vi "To Serial Form.vi"(6 "Serial Version":T1, 10 "Serializer in":refnum<class "Serializer.lvclass">, 11 "BrowerComponent in":refnum<class "BrowerComponent.lvclass">) -> (0 "error out":errorcluster, 2 "Serializer out":refnum<class "Serializer.lvclass">, 3 "BrowerComponent out":refnum<class "BrowerComponent.lvclass">)   [LabVIEW 2015, in "BrowerComponent.lvclass"]
uses:
  BrowerComponent.lvclass
  <vilib>/NI/AQ Character Lineator/Serializer/Serializer.lvclass
  <vilib>/NI/AQ Character Lineator/Serialization Common/Serial Version.ctl
  protected/ObjectAttributes.ctl
  <vilib>/NI/AQ Character Lineator/Serializable/Insert String.vi
  <vilib>/NI/AQ Character Lineator/Serializable/Insert Int32.vi
  <vilib>/NI/AQ Character Lineator/Serializer/Insert String.vi
  <vilib>/NI/AQ Character Lineator/Serializer/Insert Int32.vi
  <vilib>/NI/AQ Character Lineator/Serializer/Read Include Default Values.vi
  <vilib>/NI/AQ Character Lineator/Serializable Variant/Insert Variant.vi
  <vilib>/NI/AQ Character Lineator/Serializable/Serializable.lvclass
  <vilib>/NI/AQ Character Lineator/Serializable Variant/Serializable Variant.lvclass
  <vilib>/NI/AQ Character Lineator/Serialization Common/Serialization Common.lvlib
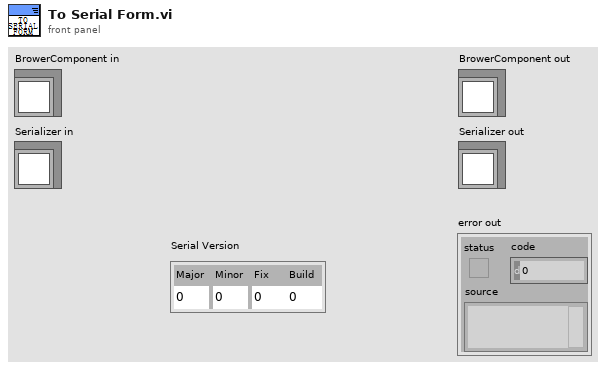
[diagram p1: front panel]
types:
  T1 = typedef "Serialization Common.lvlib/Serial Version.ctl" = cluster{"Major":u16, "Minor":u16, "Fix":u16, "Build":u16}
  T2 = typedef "BrowerComponent.lvclass/ObjectAttributes.ctl" = cluster{"ComponentID":string, "SymbolIndex":i32, "ComponentName":string, "PartsOfComponent_dict":variant}
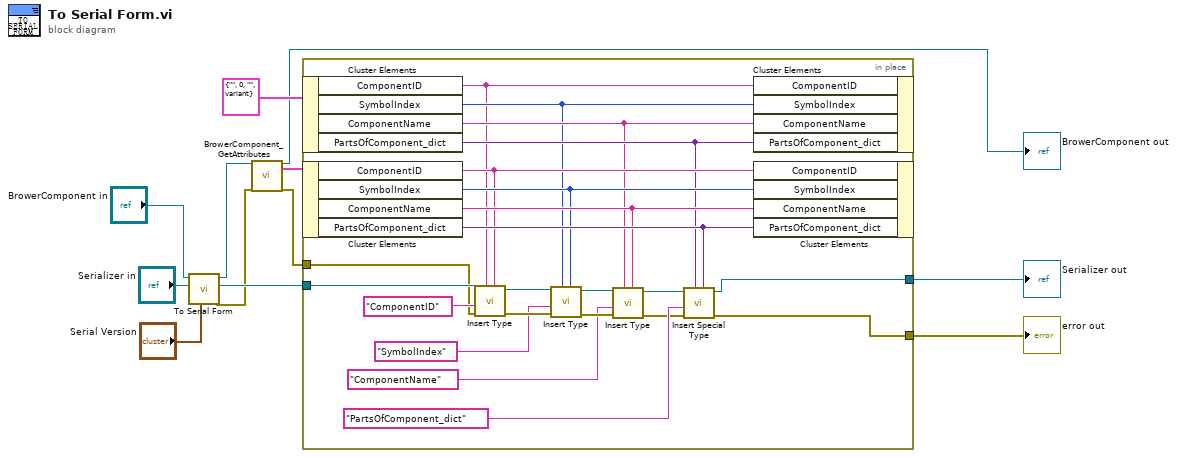
[diagram p0: block diagram]
diagram:
  n1 = call-parent "To Serial Form.vi"("Serial Version"="Serial Version", "Serializer in"="Serializer in", "Serializable in"="BrowerComponent in") -> ("error out"=w5:errorcluster, "Serializer out"=w7:refnum<class "Serializer.lvclass">, "Serializable out"=w9:refnum<class "BrowerComponent.lvclass">)  [unwired: 6 in]
  n2 = call "BrowerComponent_GetAttributes.vi"("reference in"=w9, "error in (no error)"=w5) -> ("reference out"=→"BrowerComponent out":refnum<class "BrowerComponent.lvclass">, "Data"=w8:T2, "error out"=w4:errorcluster)  [unwired: 14 in, 1 out]
  n3 = in-place {
    in-place-border: w7 -> [w33]
    in-place-border: w4 -> [w32]
    in-place-border: [w15] -> w2
    in-place-border: [w13] -> w1
    n4 = in-place-cluster #1(T2 {"ComponentID"="", "SymbolIndex"=0, "ComponentName"="", "PartsOfComponent_dict"=variant} ("Data")) -> ("ComponentID"=w17:string, "SymbolIndex"=w18:i32, "ComponentName"=w19:string, "PartsOfComponent_dict"=w20:variant)
    n5 = in-place-cluster #2(w8) -> ("ComponentID"=w21:string, "SymbolIndex"=w22:i32, "ComponentName"=w23:string, "PartsOfComponent_dict"=w24:variant)
    n6 = call-poly <vilib>:"Insert Type.vi"("String"=w21, "Default Value"=w17, "error in (no error)"=w32, "Name"="ComponentID", "Serializer in"=w33) -> ("error out"=w30:errorcluster, "Serializer out"=w31:refnum<class "Serializer.lvclass">)  [unwired: 5 in]
    n7 = call-poly <vilib>:"Insert Type.vi"("Integer"=w22, "Default Value"=w18, "error in (no error)"=w30, "Name"="SymbolIndex", "Serializer in"=w31) -> ("error out"=w27:errorcluster, "Serializer out"=w28:refnum<class "Serializer.lvclass">)  [unwired: 5 in]
    n8 = call-poly <vilib>:"Insert Type.vi"("String"=w23, "Default Value"=w19, "error in (no error)"=w27, "Name"="ComponentName", "Serializer in"=w28) -> ("error out"=w14:errorcluster, "Serializer out"=w25:refnum<class "Serializer.lvclass">)  [unwired: 5 in]
    n9 = call-poly <vilib>:"Insert Special Type.vi"("Variant"=w24, "Default Value"=w20, "error in (no error)"=w14, "Name"="PartsOfComponent_dict", "Serializer in"=w25) -> ("error out"=w13:errorcluster, "Serializer out"=w15:refnum<class "Serializer.lvclass">)  [unwired: 5 in]
    n10 = in-place-cluster #1("ComponentID"=w17, "SymbolIndex"=w18, "ComponentName"=w19, "PartsOfComponent_dict"=w20) -> ()  [unwired: 1 out]
    n11 = in-place-cluster #2("ComponentID"=w21, "SymbolIndex"=w22, "ComponentName"=w23, "PartsOfComponent_dict"=w24) -> ()  [unwired: 1 out]
  }
  "error out" <- w1
  "Serializer out" <- w2
